vi "Additive White Gaussian Noise.vi"() -> ()   [LabVIEW 2013]
uses:
  <vilib>/measure/maspectr.llb/FFT Spectrum (Mag-Phase) for 1 Chan.vi
  <vilib>/measure/NI_MABase.lvlib
  <vilib>/measure/NI_MAPro.lvlib
panel:
  in  "stop":bool
  out "Waveform Graph 2":cluster{"f0":dbl, "df":dbl, "magnitude":dbl[]}(graph)
  out "Waveform Graph":waveform(dbl)(graph)
  in  "Slide":dbl(slide) scale=0.0..10.0
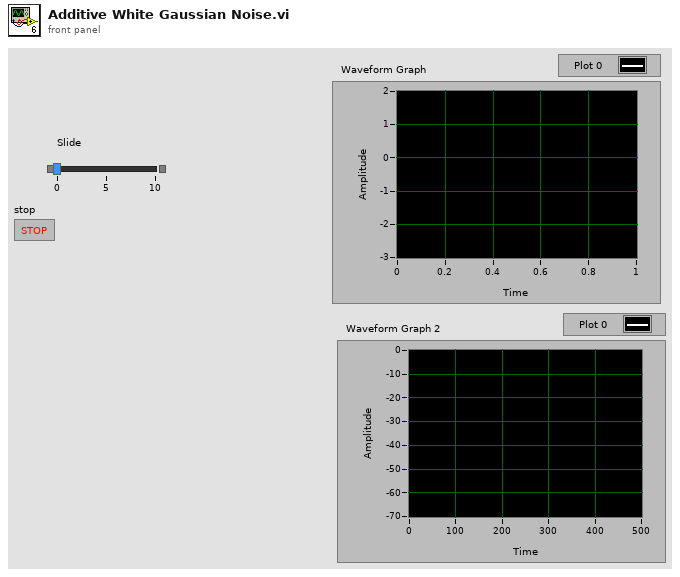
[diagram p1: front panel]
types:
  T1 = cluster{"dB On (F)":bool, "unwrap phase (F)":bool, "convert to degree (F)":bool}
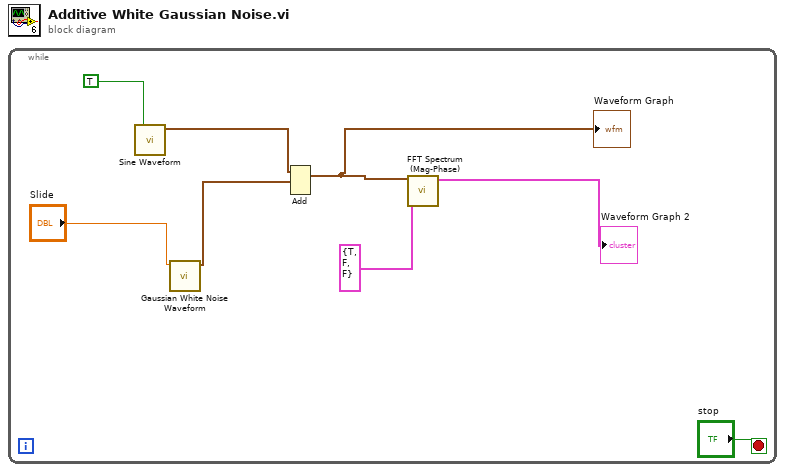
[diagram p0: block diagram]
diagram:
  n1 = while {
    stop <- "stop" stop-if-true
    n2 = call <vilib>:"Sine Waveform.vi"("reset signal"=TRUE) -> ("signal out"=w6:waveform(dbl))  [unwired: 9 in, 1 out]
    n3 = call <vilib>:"Gaussian White Noise Waveform.vi"("standard deviation"="Slide") -> ("signal out"=w5:waveform(dbl))  [unwired: 9 in, 1 out]
    n4 = Add(1:w5, 2:w6) -> (0:w2:waveform(dbl))  [unwired: 1 in, 1 out]
    "Waveform Graph" <- w2
    n5 = call-poly <vilib>:"FFT Spectrum (Mag-Phase).vi"("view"=T1 {"dB On (F)"=TRUE, "unwrap phase (F)"=FALSE, "convert to degree (F)"=FALSE}, "time signal"=w2) -> ("magnitude"=→"Waveform Graph 2":cluster{"f0":dbl, "df":dbl, "magnitude":dbl[]})  [unwired: 5 in, 4 out]
  }
